vi "Inverse Square Root.vi"(11 "Numeric":sgl=0.15625 format="%#_13g") -> (3 "Inverse Square Root":sgl)   [LabVIEW 2020, in "3D (FPGA).lvlib"]
uses:
  3D (FPGA).lvlib
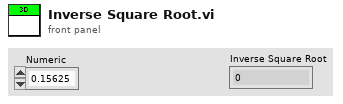
[diagram p1: front panel]
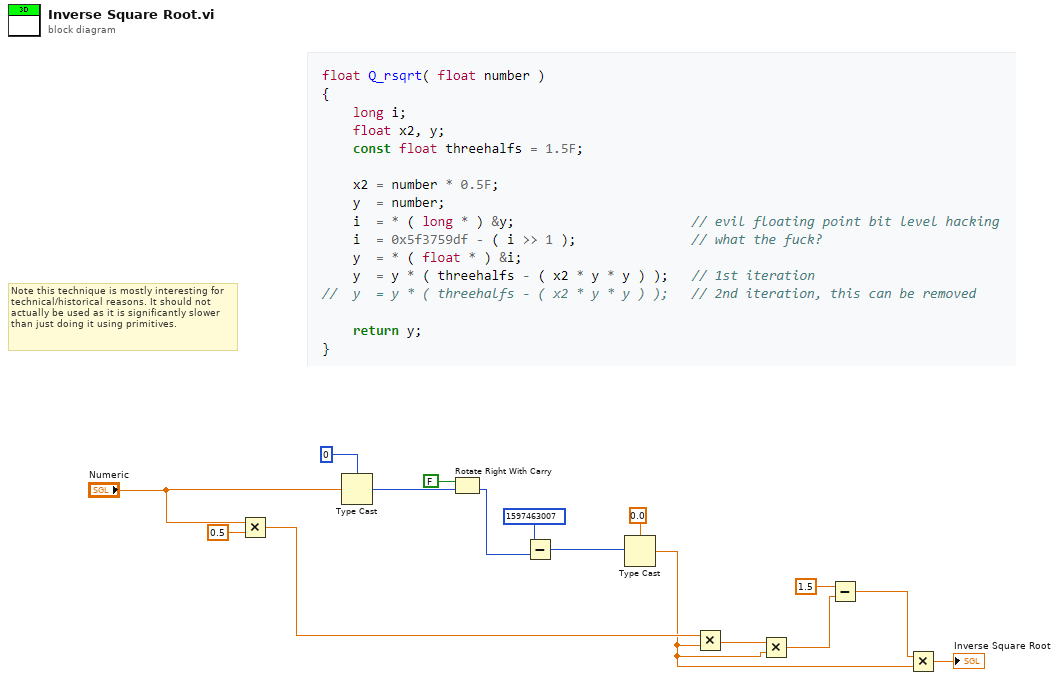
[diagram p0: block diagram]
diagram:
  # "Note this technique is mostly interesting for technical/historical reasons. It should not actually be used as it is significantly slower than just doing it using primitives."
  n1 = Multiply(x="Numeric", y=sgl 0.5) -> (x*y=w9:sgl)
  n2 = Type Cast(type=u32 0, x="Numeric") -> (*(type *) &x=w13:u32)
  n3 = Rotate Right With Carry(2:w13, 3:FALSE ("carry")) -> (0:w12:u32)  [unwired: 1 out]
  n4 = Subtract(x=u32 1597463007, y=w12) -> (x-y=w11:u32)
  n5 = Type Cast(type=sgl 0.0 ("y"), x=w11) -> (*(type *) &x=w5:sgl)
  n6 = Multiply(x=w9, y=w5) -> (x*y=w8:sgl)
  n7 = Multiply(x=w8, y=w5) -> (x*y=w6:sgl)
  n8 = Subtract(x=sgl 1.5 ("y"), y=w6) -> (x-y=w2:sgl)
  n9 = Multiply(x=w2, y=w5) -> (x*y=→"Inverse Square Root":sgl)
